vi "Recieve.vi"(8 "error in (no error)":errorcluster, 10 "Dropped?":bool, 11 "Response Core in":refnum<class "Response Core.lvclass">) -> (0 "error out":errorcluster, 1 "Success?":bool, 3 "Data":refnum<class "Data.lvclass">)   [LabVIEW 2020, in "Publisher.lvlib" / "Response Core.lvclass"]
doc: "Await the response from the sent message. Also terminates the Listen for Interrupt method when the sent message responds.\n\nThe default implementation does nothing."
uses:
  Response Core.lvclass
  PPL/HDH.Data.Generic.lvlibp/Data.lvclass
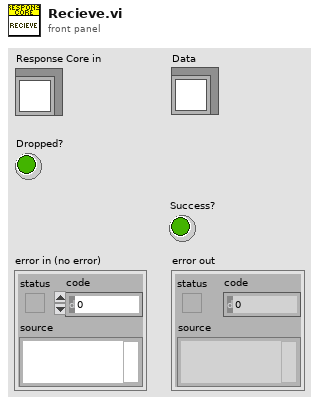
[diagram p1: front panel]
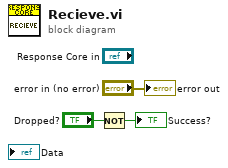
[diagram p0: block diagram]
diagram:
  n1 = Not(x="Dropped?") -> (.not. x?=→"Success?":bool)
  "error out" <- "error in (no error)"
